vi "MicroStrain 3DM-GXx Continuous Mode With Optional Measurements.vi"() -> ()   [LabVIEW 2012]
doc: "Shows how to setup the device and acquire a continuous (streaming) measurement based on the user's selected measurement type. The user is also able to request a second measurement type to be read intermittently at the user's request."
uses:
  <instrlib>/MicroStrain 3DM-GXx/Public/Data/Parse Message VIs/Parse (Euler Angles).vi
  <instrlib>/MicroStrain 3DM-GXx/Public/Data/Parse Message VIs/Parse (Delta Values).vi
  <instrlib>/MicroStrain 3DM-GXx/Public/Data/Parse Message VIs/Parse (Orientation Matrix).vi
  <instrlib>/MicroStrain 3DM-GXx/Public/Data/Parse Message VIs/Parse (Orientation Update Matrix).vi
  <instrlib>/MicroStrain 3DM-GXx/Public/Data/Parse Message VIs/Parse (Internal Device Temperature).vi
  <instrlib>/MicroStrain 3DM-GXx/Public/Data/Parse Message VIs/Parse (Acceleration, Angular Rate, And Magnetometer Vectors).vi
  <instrlib>/MicroStrain 3DM-GXx/Public/Data/Parse Message VIs/Parse (Gyro Stabilized Acceleration, Angular Rate, And Magnetometer Vectors).vi
  <instrlib>/MicroStrain 3DM-GXx/Public/Data/Parse Message VIs/Parse (Raw Acceleration And Angular Rates).vi
  <instrlib>/MicroStrain 3DM-GXx/MicroStrain 3DM-GXx.lvlib
panel:
  in  "View Output Type":u16(ring) items=["Euler Angles"=5, "DeltaAngle & DeltaVelocity"=1, "Orientation Matrix"=2, "Orientation Update Matrix"=3, "Acceleration, Angular Rate & Magnetometer Vectors"=4, "Gyro Stabilized Acceleration, Angular Rate & Magnetometer"=7, "Temperatures"=6, "Raw Accelerometer and Angular Rate"=0]
  out "Measurements":T1(tab)
  out "Raw Vector Timer":u32
  out "Raw Angular Rate Vector":sgl[](array[numeric])
  out "Raw Accelerometer Vector":sgl[](array[numeric])
  out "Delta Timer":u32
  out "Delta Velocity Vector":sgl[](array[numeric])
  out "Delta Angle Vector":sgl[](array[numeric])
  out "Orientation Matrix Timer":u32
  out "Orientation Matrix":sgl[][](array[numeric])
  out "Orientation Update Matrix Timer":u32
  out "Orientation Update Matrix":sgl[][](array[numeric])
  out "AAM Timer":u32
  out "Angular Rate":sgl[](array[numeric])
  out "Acceleration":sgl[](array[numeric])
  out "Magnetometer Vector":sgl[](array[numeric])
  out "Euler Timer":u32
  out "Yaw":sgl
  out "Pitch":sgl
  out "Roll":sgl
  out "Timer":u32
  out "Temperature":sgl
  out "GS AAM Timer":u32
  out "Gyro Stabilized Magnetometer Vetor":sgl[](array[numeric])
  out "Gyro Stabilized Angular Rate Vector":sgl[](array[numeric])
  out "Gyro Stabilized Acceleration Vector":sgl[](array[numeric])
  in  "VISA resource name":refnum<visa-resource-name>
  in  "Request Single Measurement":bool
  in  "Single Measurement Type":u16(ring) items=["Euler Angles"=5, "DeltaAngle & DeltaVelocity"=1, "Orientation Matrix"=2, "Orientation Update Matrix"=3, "Acceleration, Angular Rate & Magnetometer Vectors"=4, "Gyro Stabilized Acceleration, Angular Rate & Magnetometer"=7, "Temperatures"=6, "Raw Accelerometer and Angular Rate"=0]
  in  "Continuous Measurement Type":u16(ring) items=["Euler Angles"=5, "DeltaAngle & DeltaVelocity"=1, "Orientation Matrix"=2, "Orientation Update Matrix"=3, "Acceleration, Angular Rate & Magnetometer Vectors"=4, "Gyro Stabilized Acceleration, Angular Rate & Magnetometer"=7, "Temperatures"=6, "Raw Accelerometer and Angular Rate"=0]
  in  "Sample Rate (100 Hz)":u16=100 min=1 max=300
  in  "Stop Continuous Measurement":bool
  # "(c) 2009 - 2011 National Instruments.  ALL RIGHTS RESERVED."
  # "This VI demonstrates the procedure for a hybrid mode consisting of a continuous measurement, plus additional intermittent single measurements.\nThe device is first put into continuous mode with the selected continuous measurement type.  As data is streamed from the device the user may\nrequest a single measurement of a different type by choosing the measurement type from the 'Single Measurement Type' selector and pressing\nthe 'Request Single Measurement' button.  To change the continuous measurement type the device must be brought out of continuous mode,\nthen continuous mode must be re-initialized with the new measurement type.  This can be accomplished by pressing the stop button, choosing a\nnew continuous measurement type and then running the VI.  The user is responsible for selecting the appropriate output window from the 'View \nOutput Type' control."
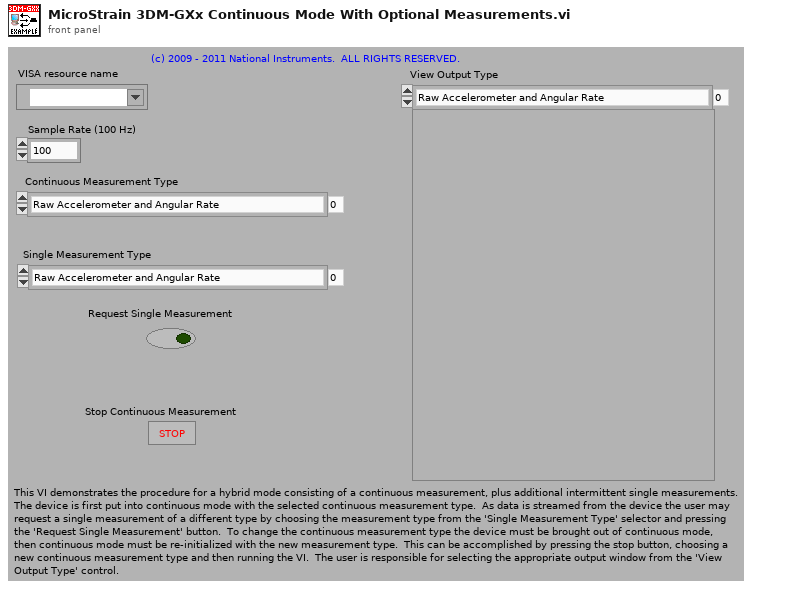
[diagram p1: front panel]
types:
  T1 = enum32{"Raw Accelerometer and Angular Rate", "Delta Angle and Delta Velocity", "Orientation Matrix", "Orientation Update Matrix", "Acceleration, Angular Rate & Magnetometer Vectors", "Euler Angles", "Temperatures", "Gyro Stabilized Acceleration, Angular Rate & Magnetometer"}
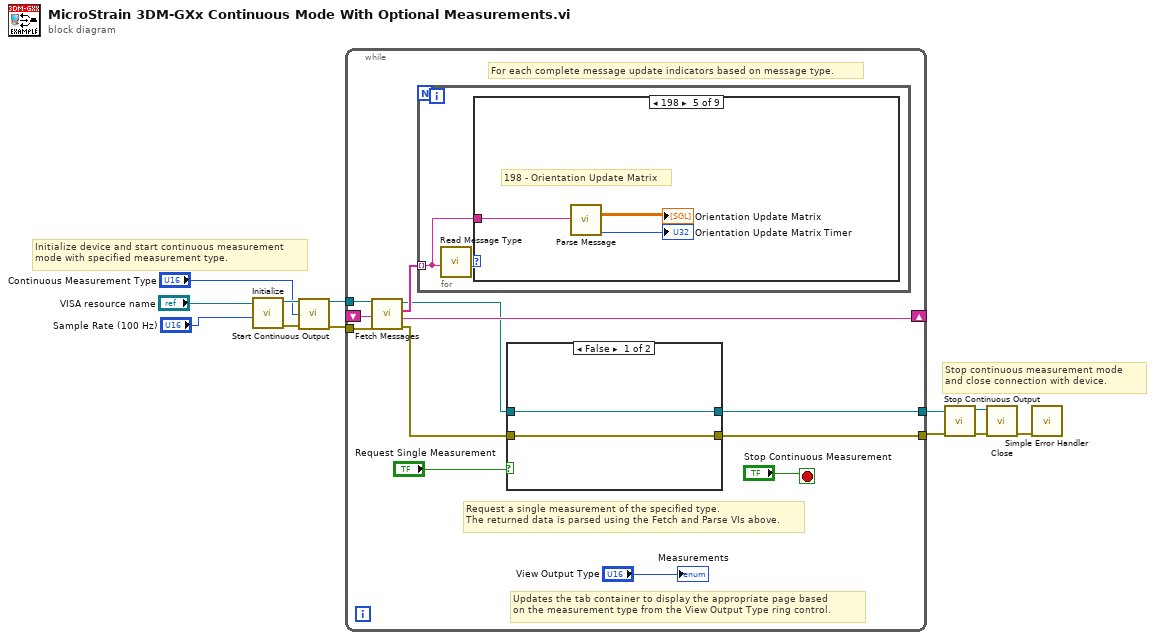
[diagram p0: block diagram]
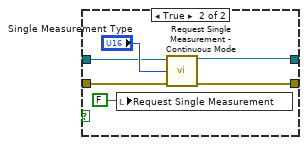
[diagram p2: hidden frame]
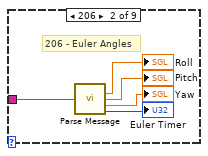
[diagram p4: hidden frame]
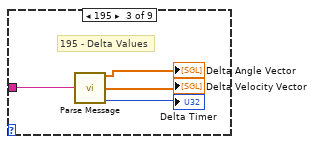
[diagram p5: hidden frame]
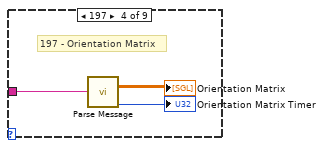
[diagram p6: hidden frame]
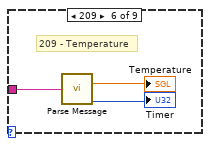
[diagram p7: hidden frame]
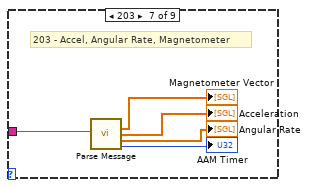
[diagram p8: hidden frame]
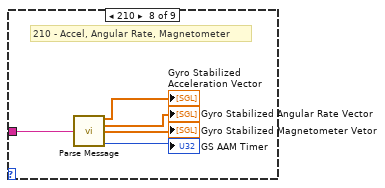
[diagram p9: hidden frame]
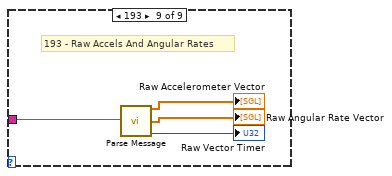
[diagram p10: hidden frame]
diagram:
  # "Stop continuous measurement mode \nand close connection with device."
  # "Initialize device and start continuous measurement \nmode with specified measurement type."
  n1 = call <instrlib>:"Initialize.vi"("Sample Rate (100 Hz)"="Sample Rate (100 Hz)", "VISA resource name"="VISA resource name") -> ("error out"=w11:errorcluster, "VISA resource name out"=w12:refnum<visa-resource-name>)  [unwired: 8 in]
  n2 = call <instrlib>:"Start Continuous Output.vi"("VISA resource name"=w12, "Continuous Measurement Type (Raw Accelerometer and Angular Rate)"="Continuous Measurement Type", "error in (no error)"=w11) -> ("VISA resource name out"=w7:refnum<visa-resource-name>, "error out"=w6:errorcluster)  [unwired: 11 in]
  n3 = while {
    tunnel: w7 -> [w24]
    tunnel: w6 -> [w23]
    shift-right: [w21] -> _
    shift-left: _ -> [w22]
    tunnel: [w15] -> w1
    tunnel: [w14] -> w2
    stop <- "Stop Continuous Measurement" stop-if-true
    # "Updates the tab container to display the appropriate page based\non the measurement type from the View Output Type ring control."
    # "Request a single measurement of the specified type.\nThe returned data is parsed using the Fetch and Parse VIs above."
    # "For each complete message update indicators based on message type."
    n4 = call <instrlib>:"Fetch Messages.vi"("error in (no error)"=w23, "Remainder In"=w22, "VISA resource name"=w24) -> ("error out"=w17:errorcluster, "Remainder Out"=w21:string, "Complete Messages"=w20:string[], "VISA resource name out"=w16:refnum<visa-resource-name>)  [unwired: 5 in]
    n5 = for {
      tunnel: w20 -> [w33] mode=indexing
      n6 = call <instrlib>:"Read Message Type.vi"("Message"=w33) -> ("Ring"=w34:u16)  [unwired: 10 in]
      n7 = case shown="198" w34 {
        tunnel: w33 -> [_ w39 w43 w46 w49 w52 w57 w62 w66]
        frame 0, Default {
          # "Unknown message type. \nDisregard message."
        }
        frame 206 {
          # "206 - Euler Angles"
          n8 = call-poly <instrlib>:"Parse Message.vi"("Message In"=w39) -> ("Roll"=→"Roll":sgl, "Pitch"=→"Pitch":sgl, "Yaw"=→"Yaw":sgl, "Timer"=→"Euler Timer":u32)  [unwired: 11 in]
        }
        frame 195 {
          # "195 - Delta Values"
          n9 = call-poly <instrlib>:"Parse Message.vi"("Message In"=w43) -> ("DeltaAngleVector"=→"Delta Angle Vector":sgl[], "DeltaVelocityVector"=→"Delta Velocity Vector":sgl[], "Timer"=→"Delta Timer":u32)  [unwired: 12 in]
        }
        frame 197 {
          # "197 - Orientation Matrix"
          n10 = call-poly <instrlib>:"Parse Message.vi"("Message In"=w46) -> ("Orientation Matrix"=→"Orientation Matrix":sgl[][], "Timer"=→"Orientation Matrix Timer":u32)  [unwired: 13 in]
        }
        frame 198 {
          # "198 - Orientation Update Matrix"
          n11 = call-poly <instrlib>:"Parse Message.vi"("Message In"=w49) -> ("Orientation Update Matrix"=→"Orientation Update Matrix":sgl[][], "Timer"=→"Orientation Update Matrix Timer":u32)  [unwired: 13 in]
        }
        frame 209 {
          # "209 - Temperature"
          n12 = call-poly <instrlib>:"Parse Message.vi"("Message In"=w52) -> ("Temperature"=→"Temperature":sgl, "Timer"=→"Timer":u32)  [unwired: 13 in]
        }
        frame 203 {
          # "203 - Accel, Angular Rate, Magnetometer"
          n13 = call-poly <instrlib>:"Parse Message.vi"("Message In"=w57) -> ("Magnetometer Vector"=→"Magnetometer Vector":sgl[], "Acceleration"=→"Acceleration":sgl[], "Angular Rate"=→"Angular Rate":sgl[], "Timer"=→"AAM Timer":u32)  [unwired: 11 in]
        }
        frame 210 {
          # "210 - Accel, Angular Rate, Magnetometer"
          n14 = call-poly <instrlib>:"Parse Message.vi"("Message In"=w62) -> ("Gyro Stabilized Acceleration Vector"=→"Gyro Stabilized Acceleration Vector":sgl[], "Gyro Stabilized Angular Rate Vector"=→"Gyro Stabilized Angular Rate Vector":sgl[], "Gyro Stabilized Magnetometer Vetor"=→"Gyro Stabilized Magnetometer Vetor":sgl[], "Timer"=→"GS AAM Timer":u32)  [unwired: 11 in]
        }
        frame 193 {
          # "193 - Raw Accels And Angular Rates"
          n15 = call-poly <instrlib>:"Parse Message.vi"("Message In"=w66) -> ("Raw Accelerometer Vector"=→"Raw Accelerometer Vector":sgl[], "Raw Angular Rate Vector"=→"Raw Angular Rate Vector":sgl[], "Timer"=→"Raw Vector Timer":u32)  [unwired: 12 in]
        }
      }
    }
    n16 = case shown="False" "Request Single Measurement" {
      tunnel: w17 -> [w25 w30]
      tunnel: w16 -> [w26 w29]
      tunnel: [w26 w28] -> w14
      tunnel: [w25 w27] -> w15
      frame False {
      }
      frame True {
        n17 = local write "Request Single Measurement"(FALSE ("Request Measurement")) -> ()
        n18 = call <instrlib>:"Request Single Measurement - Continuous Mode.vi"("VISA resource name"=w29, "Single Measurement Type (Raw Accelerometer and Angular Rate)"="Single Measurement Type", "error in (no error)"=w30) -> ("VISA resource name out"=w28:refnum<visa-resource-name>, "error out"=w27:errorcluster)  [unwired: 11 in]
      }
    }
    "Measurements" <- "View Output Type"
  }
  n19 = call <instrlib>:"Stop Continuous Output.vi"("error in (no error)"=w1, "VISA resource name"=w2) -> ("error out"=w5:errorcluster, "VISA resource name out"=w4:refnum<visa-resource-name>)  [unwired: 8 in]
  n20 = call <instrlib>:"Close.vi"("error in (no error)"=w5, "VISA resource name"=w4) -> ("error out"=w3:errorcluster)  [unwired: 9 in]
  n21 = call <vilib>:"Simple Error Handler.vi"("error in (no error)"=w3) -> ()  [unwired: 4 in, 5 out]
